vi "Read Unit Yaw-Pitch-Roll.vi"(11 "PigeonIMUDevRef":T3 {"Type" items=["CAN"=352321536, "TalonSRX"=33554432]}) -> (2 "Unit Yaw-Pitch-Roll Out":T1 {"Roll" scale format="%.3f"; "Pitch" scale format="%.3f"; "Yaw" scale format="%.3f"}, 3 "PigeonIMUDevRef Out":T3 {"Type" items=["CAN"=352321536, "TalonSRX"=33554432]}, 5 "Yaw Pitch Roll Out":T5)   [LabVIEW 2020, in "PigeonIMU_SEN.lvlib"]
uses:
  PigeonIMU_SEN.lvlib
  <vilib>/Rock Robotics/WPI/ThirdParty/Phoenix-LabVIEW/Pigeon IMU/CTRE_PigeonIMU_DeviceRef.ctl
  <vilib>/Rock Robotics/WPI/ThirdParty/Phoenix-LabVIEW/Pigeon IMU/CTRE_PigeonIMU_ConnectionType.ctl
  Shared Code/TypeDefs/Cluster_Unity Yaw-Pitch-Roll.ctl
  Shared Code/TypeDefs/Dial_Compase heading unit circle CCW positive.ctl
  <vilib>/Rock Robotics/WPI/ThirdParty/Phoenix-LabVIEW/Pigeon IMU/CTRE_PigeonIMU_GetYPR.vi
  Type Defs/Cluster_Yaw Pitch Roll in Deg.ctl
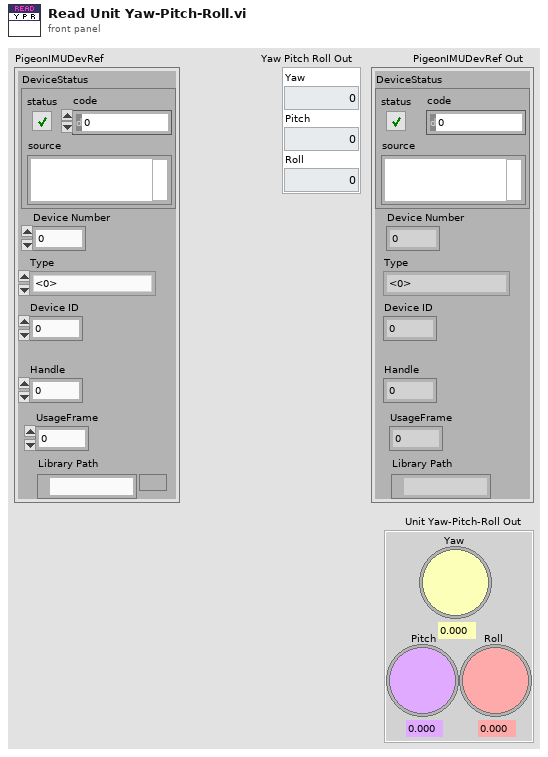
[diagram p1: front panel]
types:
  T1 = typedef "Cluster_Unity Yaw-Pitch-Roll.ctl" = cluster{"Yaw":T2, "Pitch":T2, "Roll":T2}
  T2 = typedef "Dial_Compase heading unit circle CCW positive.ctl" = dbl
  T3 = typedef "CTRE_PigeonIMU_DeviceRef.ctl" = cluster{"DeviceStatus":errorcluster, "Device Number":u8, "Type":T4, "Device ID":u32, "Handle":u64, "UsageFrame":u32, "Library Path":path}
  T4 = typedef "CTRE_PigeonIMU_ConnectionType.ctl" = u32
  T5 = typedef "Cluster_Yaw Pitch Roll in Deg.ctl" = cluster{"Yaw":dbl, "Pitch":dbl, "Roll":dbl}
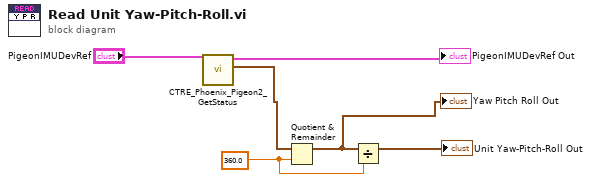
[diagram p0: block diagram]
diagram:
  w2 = 360.0
  n1 = call-poly <vilib>:"CTRE_Phoenix_Pigeon2_GetStatus.vi"("PigeonIMUDevRef"="PigeonIMUDevRef") -> ("Yaw Pitch Roll"=w4:cluster{"Yaw":dbl, "Pitch":dbl, "Roll":dbl}, "PigeonIMUDevRef"=→"PigeonIMUDevRef Out":T3)  [unwired: 8 in, 1 out]
  n2 = Quotient & Remainder(x=w4, y=w2) -> (x-y*floor(x/y)=w1:cluster{"Yaw":dbl, "Pitch":dbl, "Roll":dbl})  [unwired: 1 out]
  "Yaw Pitch Roll Out" <- w1
  n3 = Divide(x=w1, y=w2) -> (x/y=→"Unit Yaw-Pitch-Roll Out":cluster{"Yaw":dbl, "Pitch":dbl, "Roll":dbl})
